vi "rotate2DArray.vi"(1 "Direction (clockwise)":enum16{"clockwise", "counter-clockwise"}(ring), 2 "Array":u32[][](array[numeric])) -> (0 "Rotated Array":u32[][](array[numeric]))   [LabVIEW 2013]
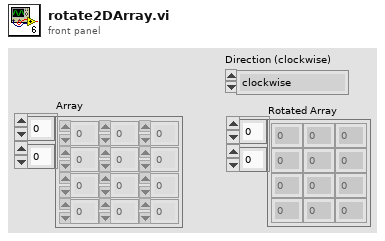
[diagram p1: front panel]
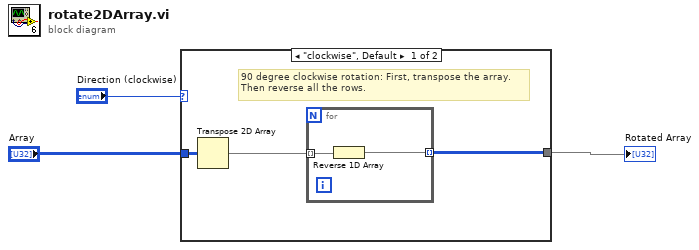
[diagram p0: block diagram]
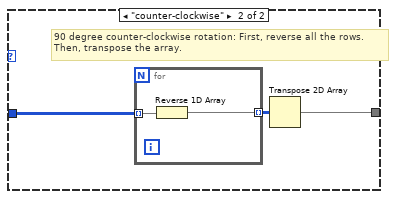
[diagram p2: hidden frame]
diagram:
  n1 = case shown="\"clockwise\", Default" "Direction (clockwise)" {
    tunnel: "Array" -> [w6 w9]
    tunnel: [w4 w10] -> w2
    frame "clockwise", Default {
      # "90 degree clockwise rotation: First, transpose the array.\nThen reverse all the rows."
      n2 = Transpose 2D Array(2D array=w6) -> (transposed array=w5:u32[][])
      n3 = for {
        tunnel: w5 -> [w8] mode=indexing
        tunnel: [w7] -> w4 mode=indexing
        n4 = Reverse 1D Array(array=w8) -> (reversed array=w7:u32[])
      }
    }
    frame "counter-clockwise" {
      # "90 degree counter-clockwise rotation: First, reverse all the rows.\nThen, transpose the array."
      n5 = for {
        tunnel: w9 -> [w13] mode=indexing
        tunnel: [w12] -> w11 mode=indexing
        n6 = Reverse 1D Array(array=w13) -> (reversed array=w12:u32[])
      }
      n7 = Transpose 2D Array(2D array=w11) -> (transposed array=w10:u32[][])
    }
  }
  "Rotated Array" <- w2
